vi "Read Stunt.vi"(8 "error in":errorcluster, 11 "Path":path) -> (0 "error out":errorcluster, 3 "Array":i32[][](array[numeric]))   [LabVIEW 2019, in "flashcards.lvlib"]
uses:
  flashcards.lvlib
  Colors.ctl
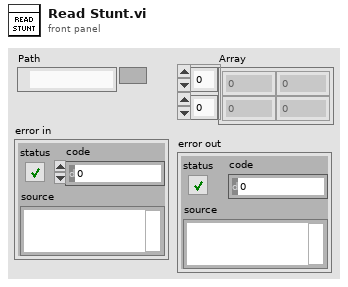
[diagram p1: front panel]
types:
  T1 = typedef "flashcards.lvlib/Colors.ctl" = enum16{"Black", "White", "Orange", "Red", "Blue", "Green", "None"}
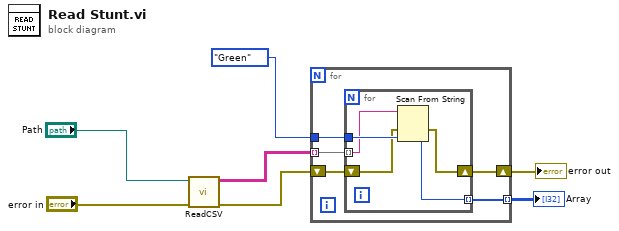
[diagram p0: block diagram]
diagram:
  n1 = call "ReadCSV.vi"("error in (no error)"="error in", "file path"="Path") -> ("error out"=w2:errorcluster, "Data"=w6:string[][])  [unwired: 8 in]
  n2 = for {
    tunnel: [w12] -> w7 mode=indexing
    tunnel: w6 -> [w11] mode=indexing
    tunnel: Colors."Green" ("Color") -> [w10]
    shift-right: [w8] -> w1
    shift-left: w2 -> [w9]
    n3 = for {
      tunnel: [w13] -> w12 mode=indexing
      tunnel: w11 -> [w16] mode=indexing
      tunnel: w10 -> [w17]
      shift-right: [w14] -> w8
      shift-left: w9 -> [w15]
      n4 = Scan From String(input string=w16, error in=w15, default 1=w17) -> (error out=w14:errorcluster, output 1=w13:T1)  [unwired: 2 in, 2 out]
    }
  }
  "Array" <- w7
  "error out" <- w1
